vi "DriverStation Get Mode And Status.vi"() -> (0 "OutputsEnabled?":bool, 2 "Match Time(s)":sgl, 3 "currentOpMode":u64, 4 "details":T1)   [LabVIEW 2026, in "MrcLib.lvlib"]
doc: "This VI returns the operating mode and status of the robot."
uses:
  MrcLib.lvlib
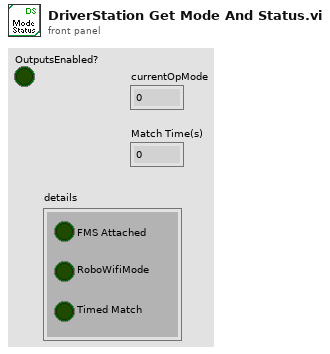
[diagram p1: front panel]
types:
  T1 = cluster{"FMS Attached":bool, "RoboWifiMode":bool, "Timed Match":bool}
  T2 = typedef "MrcLib.lvlib/MRC_ControlData.ctl" = cluster{"controlFlags":u32, "matchTime":u16, "currentOpMode":u64, "gameDataLength":u8, "gameData":cluster{"gameData 0":u8, "gameData 1":u8, "gameData 2":u8, "gameData 3":u8, "gameData 4":u8, "gameData 5":u8, "gameData 6":u8, "gameData 7":u8}}
  T3 = cluster{"FMSConnected":bool, "SupportOpModes":bool, "Alliance":u32, "RoboWifiMode":bool, "Timed Match":bool}
  T4 = cluster{"FMSConnected":bool, "RoboWifiMode":bool, "Timed Match":bool}
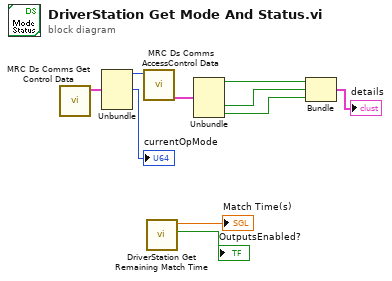
[diagram p0: block diagram]
diagram:
  n1 = call "MRC Ds Comms Get Control Data.vi"() -> ("data out"=w9:T2)  [unwired: 10 in, 1 out]
  n2 = Unbundle(w9) -> ("controlFlags"=w8:u32, "currentOpMode"=→"currentOpMode":u64)  [unwired: 3 out]
  n3 = call "MRC Ds Comms AccessControl Data.vi"("controlFlag"=w8) -> ("info"=w10:T3)  [unwired: 7 in, 3 out]
  n4 = call "DriverStation Get Remaining Match Time.vi"() -> ("OutputsEnabled?"=→"OutputsEnabled?":bool, "Match Time(s)"=→"Match Time(s)":sgl)  [unwired: 9 in, 1 out]
  n5 = Unbundle(w10) -> ("FMSConnected"=w6:bool, "RoboWifiMode"=w5:bool, "Timed Match"=w4:bool)  [unwired: 2 out]
  n6 = Bundle("FMSConnected"=w6, "RoboWifiMode"=w5, "Timed Match"=w4) -> (→"details":T4)  [unwired: 1 in]
